vi "LangTag to Code Page Lookup.vi"(11 "Tag":string) -> (3 "Language":T1, 5 "Found?":bool)   [LabVIEW 2013, in "SET Project Data.lvlib"]
uses:
  SET Project Data.lvlib
  Types/ProjFile_Language Entry.ctl
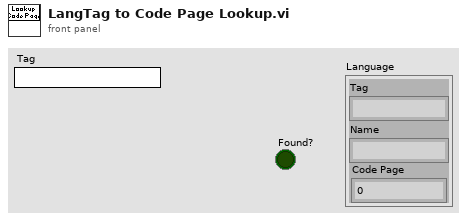
[diagram p1: front panel]
types:
  T1 = typedef "SET Project Data.lvlib/ProjFile_Language Entry.ctl" = cluster{"Tag":string, "Name":string, "Code Page":u16}
  T2 = cluster{"Name":string, "Tag":string, "Code Page":u16}[]
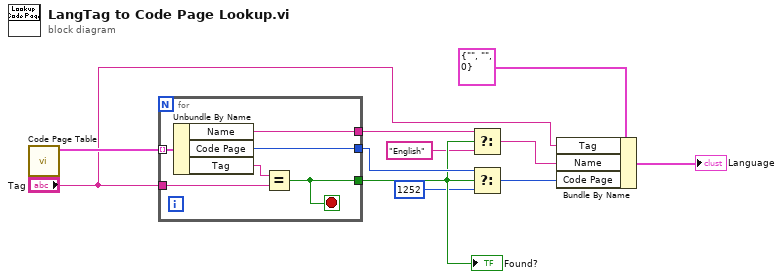
[diagram p0: block diagram]
diagram:
  n1 = call "Code Page Table.vi"() -> ("Code Page Table"=w11:T2)  [unwired: 11 in]
  n2 = for {
    tunnel: w11 -> [w17] mode=indexing
    tunnel: "Tag" -> [w16]
    tunnel: [w14] -> w8
    tunnel: [w13] -> w10
    tunnel: [w12] -> w9
    stop <- w14 stop-if-true
    n3 = Unbundle By Name(w17) -> ("Name"=w13:string, "Code Page"=w12:u16, "Tag"=w15:string)
    n4 = Equal?(x=w15, y=w16) -> (x = y?=w14:bool)
  }
  "Found?" <- w8
  n5 = Select(t=w10, s=w8, f="English") -> (s? t:f=w2:string)
  n6 = Select(t=w9, s=w8, f=u16 1252) -> (s? t:f=w3:u16)
  n7 = Bundle By Name(cluster=T1 {"Tag"="", "Name"="", "Code Page"=0} ("Language"), "Tag"="Tag", "Name"=w2, "Code Page"=w3) -> (→"Language":T1)
